vi "UDP Data Logger.vi"() -> ()   [LabVIEW 2012]
doc: "Use this VI with the UDP Sender VI. Run this VI first.\n\nThe UDP protocol differs from TCP in that there is no error-checking with the packets of information that are sent, and thus no guarantee whatsoever that an intended recipient will actually receive a given piece of data.\n\nUDP does offer the ability to \"broadcast\" data across a network--simply specify an IP Address of all ones (255.255.255.255) to attempt to broadcast information network-wide. Keep in mind that routers and other network hardware will generally refuse to forward the broadcast beyond certain points, so the extent of the broadcast will in practice be limited."
uses:
  <vilib>/vision/Image Controls.llb/IMAQ Image.ctl
panel:
  out "Attitude Status":T1
  out "Objects":T2(array[cluster])
  in  "Object Data Downlinked?":bool
  out "Fame Rate (fps)":dbl
  out "Data Rate (kb/s)":dbl
  out "Image Out":T3(plugin-control)
  in  "Port":u16=61557
  in  "stop":bool
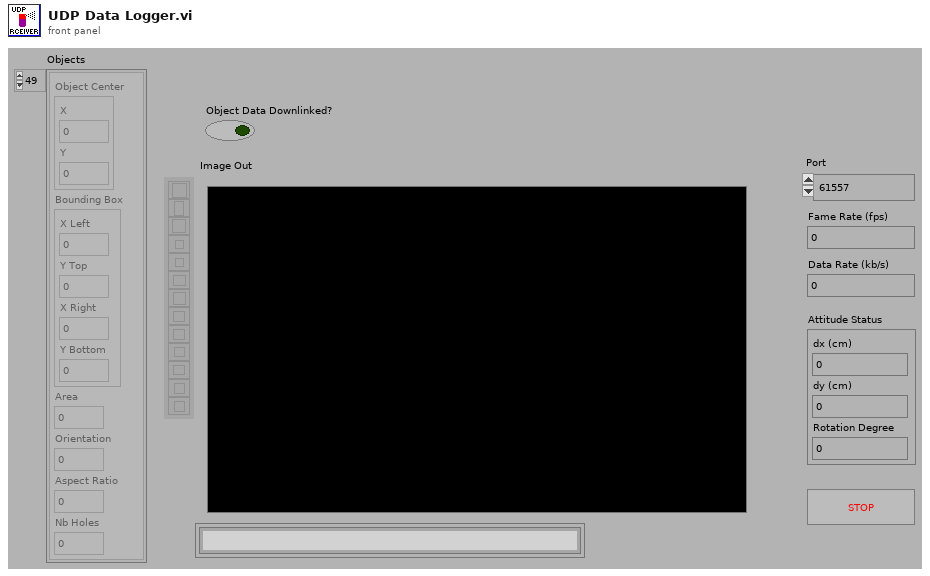
[diagram p1: front panel]
types:
  T1 = cluster{"dx (cm)":dbl, "dy (cm)":dbl, "Rotation Degree":dbl}
  T2 = cluster{"Object Center":cluster{"X":sgl, "Y":sgl}, "Bounding Box":cluster{"X Left":i32, "Y Top":i32, "X Right":i32, "Y Bottom":i32}, "Area":sgl, "Orientation":sgl, "Aspect Ratio":sgl, "Nb Holes":i32}[]
  T3 = typedef "IMAQ Image.ctl" = refnum<image>
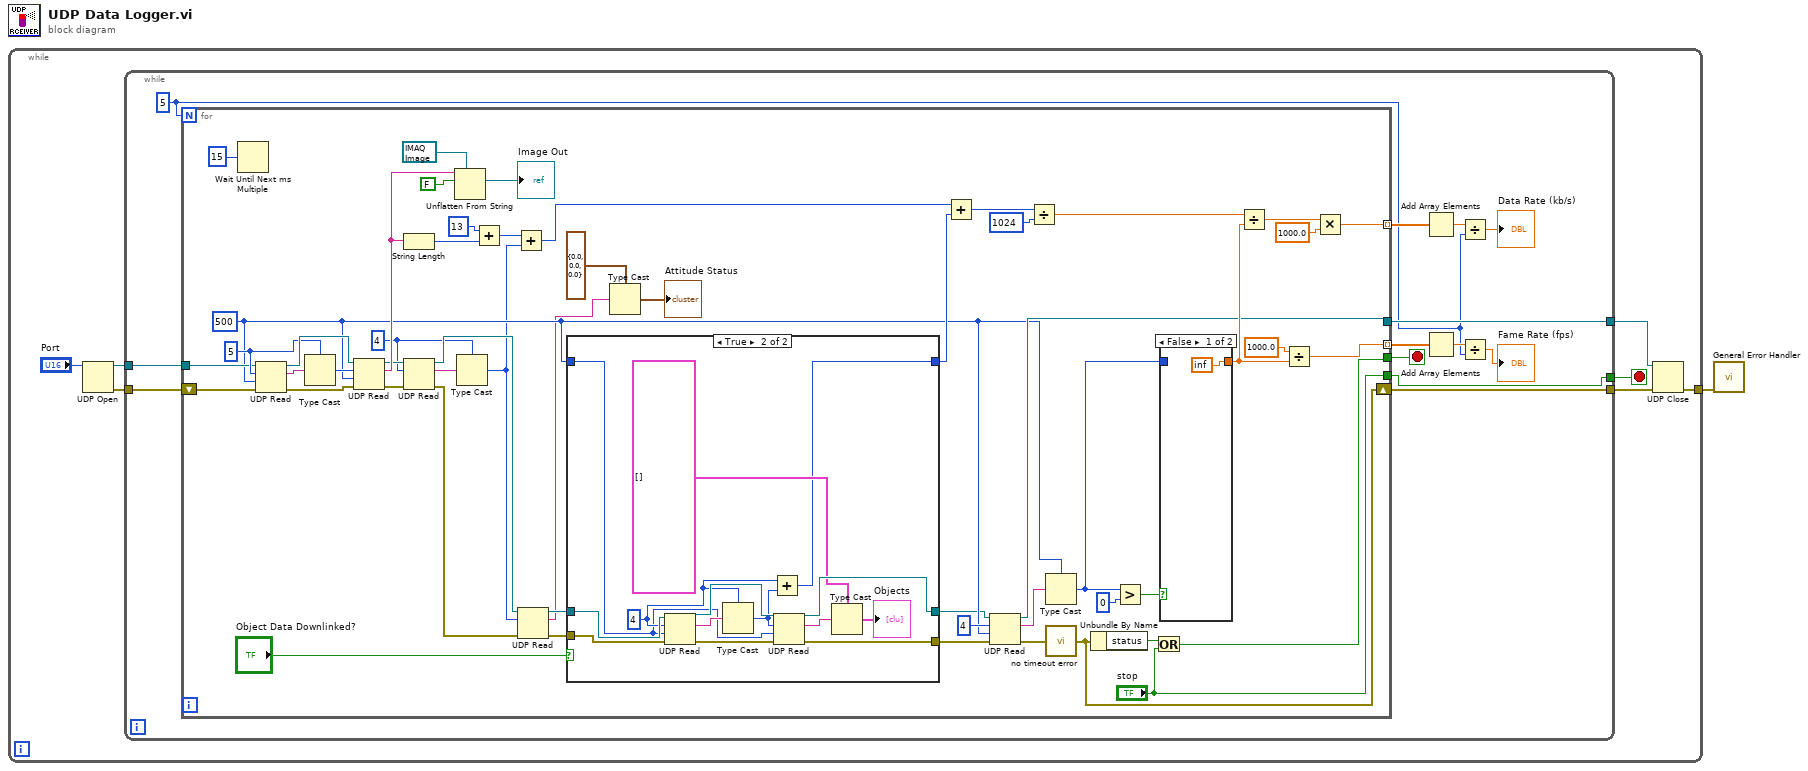
[diagram p0: block diagram]
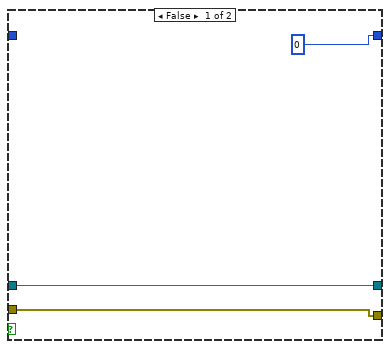
[diagram p2: hidden frame]
diagram:
  n1 = while {
    tunnel: [w2] -> w1
    stop <- w5 stop-if-true
    n2 = UDP Open(11:"Port") -> (port=w6:refnum<k16>, 0:w7:errorcluster)  [unwired: 4 in, 1 out]
    n3 = while {
      tunnel: w7 -> [w21]
      tunnel: w6 -> [w20]
      tunnel: [w19] -> w5
      tunnel: [w14] -> w4
      tunnel: [w13] -> w3
      stop <- w15 stop-if-true
      w10 = 5
      n4 = for {
        N: w10 -> [_]
        tunnel: [w39] -> w13
        tunnel: w20 -> [w55]
        shift-left: w21 -> [w54]
        shift-right: [w73] -> w14
        tunnel: ["stop"] -> w19
        tunnel: [w51] -> w18 mode=indexing
        tunnel: [w50] -> w15
        tunnel: [w49] -> w12 mode=indexing
        w28 = 4 ("max size (548)")
        w60 = 5 ("max size (548)")
        w37 = 500
        n5 = Wait Until Next ms Multiple(millisecond multiple=u32 15) -> ()  [unwired: 1 out]
        n6 = UDP Read(connection ID=w55, max size (548)=w60, timeout ms (25000)=w37, 8:w54) -> (data out=w62:string, error out=w67:errorcluster, 3:w68:refnum<k16>)  [unwired: 2 out]
        n7 = Type Cast(type=w60, x=w62) -> (*(type *) &x=w61:i32)
        n8 = UDP Read(connection ID=w68, max size (548)=w61, timeout ms (25000)=w37, 8:w67) -> (data out=w69:string, error out=w34:errorcluster, 3:w35:refnum<k16>)  [unwired: 2 out]
        n9 = String Length(string=w69) -> (length=w46:i32)
        n10 = UDP Read(connection ID=w35, max size (548)=w28, 8:w34) -> (data out=w29:string, error out=w31:errorcluster, 3:w33:refnum<k16>)  [unwired: 1 in, 2 out]
        n11 = Unflatten From String(type=T3 refnum ("Image Out"), binary string=w69, data includes array or string size? (T)=FALSE) -> (value=→"Image Out":T3)  [unwired: 2 in, 2 out]
        n12 = Type Cast(type=w28, x=w29) -> (*(type *) &x=w23:i32)
        n13 = Add(x=13, y=w46) -> (x+y=w24:i32)
        n14 = Add(x=w24, y=w23) -> (x+y=w22:i32)
        n15 = UDP Read(connection ID=w33, max size (548)=w23, 8:w31) -> (data out=w27:string, error out=w30:errorcluster, 3:w32:refnum<k16>)  [unwired: 1 in, 2 out]
        n16 = case shown="True" "Object Data Downlinked?" {
          tunnel: [w77 w86] -> w36
          tunnel: w32 -> [w77 w88]
          tunnel: [w76 w89] -> w41
          tunnel: w30 -> [w76 w91]
          tunnel: [0 w80] -> w43
          tunnel: w37 -> [_ w78]
          frame False {
          }
          frame True {
            w79 = 4 ("max size (548)")
            n17 = UDP Read(connection ID=w88, max size (548)=w79, timeout ms (25000)=w78, 8:w91) -> (data out=w85:string, error out=w90:errorcluster, 3:w87:refnum<k16>)  [unwired: 2 out]
            n18 = Type Cast(type=w79, x=w85) -> (*(type *) &x=w81:i32)
            n19 = Add(x=w79, y=w81) -> (x+y=w80:i32)
            n20 = UDP Read(connection ID=w87, max size (548)=w81, timeout ms (25000)=w78, 8:w90) -> (data out=w83:string, error out=w89:errorcluster, 3:w86:refnum<k16>)  [unwired: 2 out]
            n21 = Type Cast(type=T2 [] ("Objects"), x=w83) -> (*(type *) &x=→"Objects":T2)
          }
        }
        n22 = Type Cast(type=cluster{"dx":dbl, "dy":dbl, "FOG Degree":dbl} {"dx"=0.0, "dy"=0.0, "FOG Degree"=0.0} ("output cluster"), x=w27) -> (*(type *) &x=→"Attitude Status":cluster{"dx":dbl, "dy":dbl, "FOG Degree":dbl})
        n23 = Add(x=w22, y=w43) -> (x+y=w44:i32)
        n24 = UDP Read(connection ID=w36, max size (548)=4, timeout ms (25000)=w37, 8:w41) -> (data out=w38:string, error out=w40:errorcluster, 3:w39:refnum<k16>)  [unwired: 2 out]
        n25 = Divide(x=w44, y=1024) -> (x/y=w66:dbl)
        n26 = Type Cast(type=w37, x=w38) -> (*(type *) &x=w56:i32)
        n27 = call "no timeout error.vi"("error in (no error)"=w40) -> ("error out"=w73:errorcluster)
        n28 = Unbundle By Name(w73) -> ("status"=w74:bool)
        n29 = Greater?(x=w56, y=0) -> (0:w57:bool)
        n30 = Or(x=w74, y="stop") -> (x .or. y?=w50:bool)
        n31 = case shown="False" w57 {
          tunnel: [inf w93] -> w53
          tunnel: w56 -> [_ w93]
          frame False {
          }
          frame True {
          }
        }
        n32 = Divide(x=w66, y=w53) -> (x/y=w65:dbl)
        n33 = Divide(x=1000.0, y=w53) -> (x/y=w49:dbl)
        n34 = Multiply(x=w65, y=1000.0) -> (x*y=w51:dbl)
      }
      n35 = Add Array Elements(numeric array=w18) -> (sum=w16:dbl)
      n36 = Add Array Elements(numeric array=w12) -> (sum=w11:dbl)
      n37 = Divide(x=w16, y=w10) -> (x/y=→"Data Rate (kb/s)":dbl)
      n38 = Divide(x=w11, y=w10) -> (x/y=→"Fame Rate (fps)":dbl)
    }
    n39 = UDP Close(connection ID=w3, 8:w4) -> (error out=w2:errorcluster)  [unwired: 1 out]
  }
  n40 = call <vilib>:"General Error Handler.vi"("error in (no error)"=w1) -> ()  [unwired: 10 in, 5 out]
